vi "Example Shift Register Loop 1.vi"(8 "Error In":errorcluster, 10 "userString1":string, 11 "numberA":dbl) -> (0 "Error Out":errorcluster)   [LabVIEW 2014]
panel:
  out "userString1 2":string
  out "numberA 2":dbl
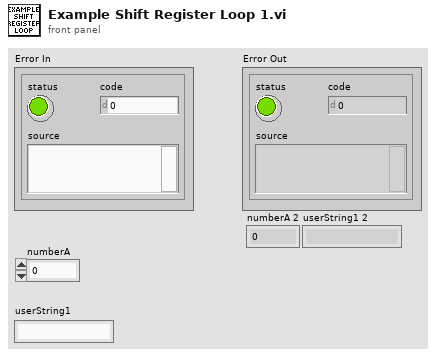
[diagram p1: front panel]
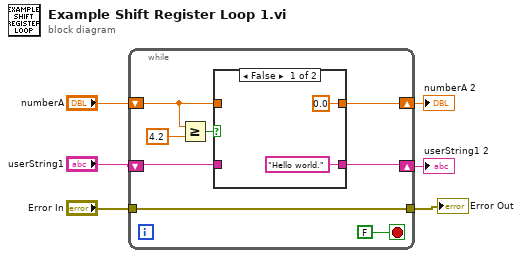
[diagram p0: block diagram]
diagram:
  n1 = while {
    tunnel: [w14] -> w6
    tunnel: "Error In" -> [w14]
    shift-right: [w7] -> w3
    shift-left: "numberA" -> [w11]
    shift-right: [w10] -> w2
    shift-left: "userString1" -> [w9]
    stop <- FALSE stop-if-true
    n2 = Greater Or Equal?(x=w11, y=4.2) -> (x >= y?=w13:bool)
    n3 = case shown="False" w13 {
      tunnel: [0.0 ("numberA") w18] -> w7
      tunnel: w11 -> [_ w18]
      tunnel: ["Hello world." ("userString1") w17] -> w10
      tunnel: w9 -> [_ w17]
      frame False {
      }
      frame True {
      }
    }
  }
  "Error Out" <- w6
  "numberA 2" <- w3
  "userString1 2" <- w2
